vi "Hi-Tec_Voltage_calculator.vi"(0 "Carrier_1 Q (l/min)":dbl=20.0 format="%.2f", 2 "Mode":enum16{"Control Hi-Tec", "Check Hi-Tec Demands"}(ring), 5 "Carrier_2 Q (l/min)":dbl=20.0 format="%.2f", 7 "Trace Q (l/min)":dbl=20.0 format="%.2f", 9 "Release temp (deg C)":dbl=20.0 format="%.2f", 11 "Atmos Pres (mbars)":dbl=1000.0 format="%.2f", 12 "Carrier Info":string) -> (4 "Carrier 1 Voltage":dbl format="%.3f", 6 "Carrier 2 Voltage":dbl format="%.2f", 8 "Trace Voltage":dbl format="%.2f", 10 "Flowrates (kg/min)":dbl[](array[numeric]) format="%.2f", 14 "Trace_2 Voltage":dbl format="%.2f", 15 "Error Comments":string)   [LabVIEW 2015]
uses:
  Anemometry/Anemometry Sub Vis/Globals/Gas_management_global.vi
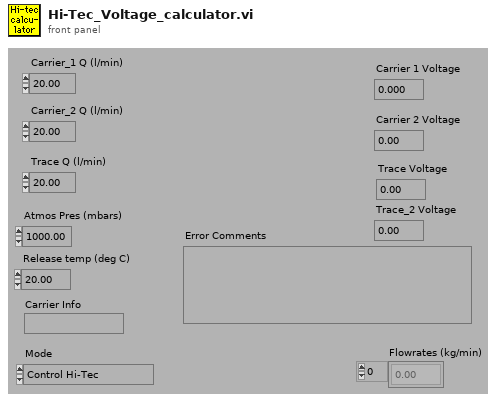
[diagram p1: front panel]
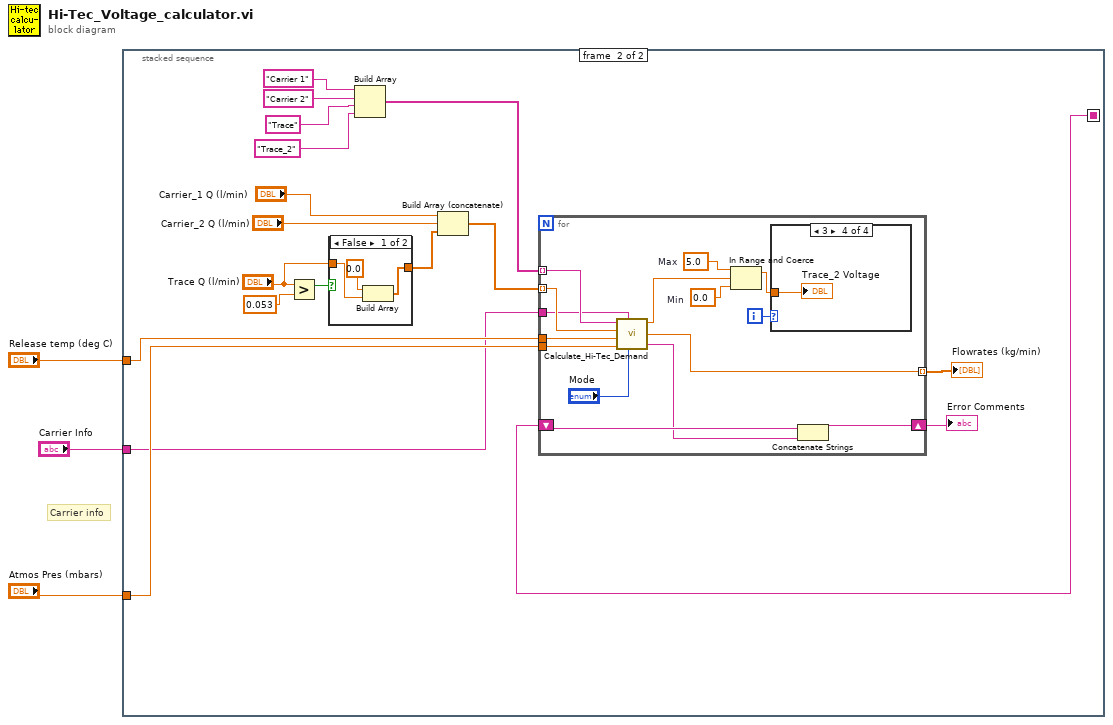
[diagram p0: block diagram]
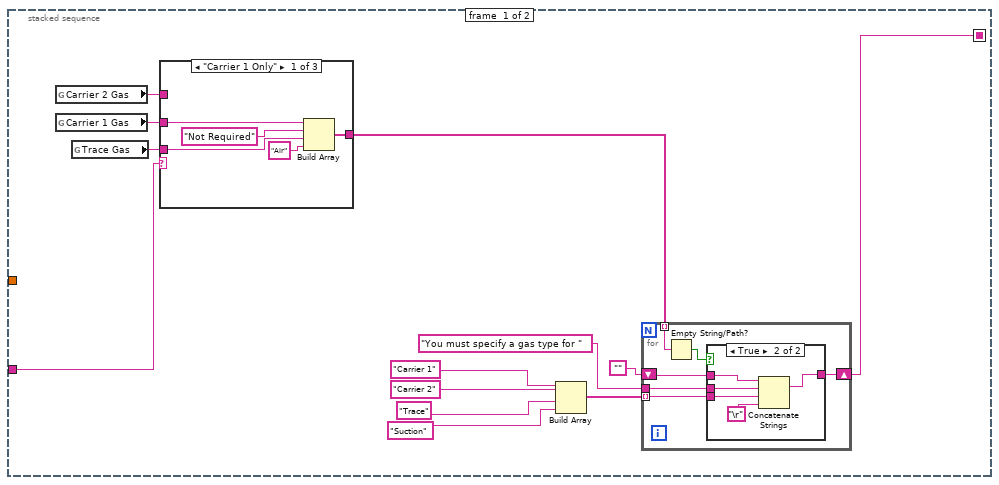
[diagram p2: hidden frame]
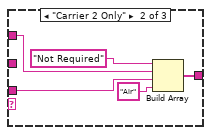
[diagram p4: hidden frame]
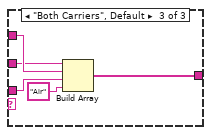
[diagram p5: hidden frame]
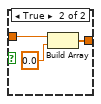
[diagram p6: hidden frame]
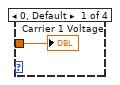
[diagram p7: hidden frame]
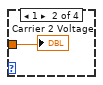
[diagram p8: hidden frame]
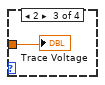
[diagram p9: hidden frame]
diagram:
  # "Carrier info"
  n1 = stacked-sequence {
    seq-local: [w6 _] -> [_ w58]
    tunnel: "Release temp (deg C)" -> [_ w60]
    tunnel: "Atmos Pres (mbars)" -> [_ w61]
    tunnel: "Carrier Info" -> [w4 w56]
    frame #0 {
      n2 = global read "Gas_management_global.vi" "Carrier 2 Gas"() -> (w14:string)
      n3 = global read "Gas_management_global.vi" "Carrier 1 Gas"() -> (w16:string)
      n4 = global read "Gas_management_global.vi" "Trace Gas"() -> (w15:string)
      n5 = case shown="\"Carrier 1 Only\"" w4 {
        tunnel: [w31 w36 w42] -> w7
        tunnel: w16 -> [w30 _ w39]
        tunnel: w15 -> [w29 w34 w41]
        tunnel: w14 -> [_ w35 w40]
        frame "Carrier 1 Only" {
          n6 = Build Array(w30, "Not Required" ("Input Element"), w29, "Air") -> (w31:string[])
        }
        frame "Carrier 2 Only" {
          n7 = Build Array("Not Required" ("Input Element"), w35, w34, "Air") -> (w36:string[])
        }
        frame "Both Carriers", Default {
          n8 = Build Array(w39, w40, w41, "Air") -> (w42:string[])
        }
      }
      n9 = Build Array("Carrier 1" ("Gas Line Name"), "Carrier 2" ("Gas Line Name"), "Trace" ("Gas Line Name"), "Suction" ("Gas Line Name")) -> (w13:string[])
      n10 = for {
        shift-right: [w18] -> w6
        shift-left: "" -> [w19]
        tunnel: "You must specify a gas type for " -> [w21]
        tunnel: w13 -> [w20] mode=indexing
        tunnel: w7 -> [w17] mode=indexing
        n11 = Empty String/Path?(string/path=w17) -> (empty?=w22:bool)
        n12 = case shown="True" w22 {
          tunnel: w21 -> [_ w28]
          tunnel: w20 -> [_ w27]
          tunnel: w19 -> [w23 w26]
          tunnel: [w23 w25] -> w18
          frame False {
          }
          frame True {
            n13 = Concatenate Strings(w26, w28, w27, "\r") -> (w25:string)
          }
        }
      }
    }
    frame #1 {
      n14 = Greater?(x="Trace Q (l/min)", y=0.053) -> (0:w46:bool)
      n15 = case shown="False" w46 {
        tunnel: "Trace Q (l/min)" -> [w63 w67]
        tunnel: [w64 w65] -> w44
        frame False {
          n16 = Build Array(0.0 ("element"), w63) -> (w64:dbl[])
        }
        frame True {
          n17 = Build Array(w67, 0.0 ("element")) -> (w65:dbl[])
        }
      }
      n18 = Build Array("Carrier 1" ("Gas Line Name"), "Carrier 2" ("Gas Line Name"), "Trace" ("Gas Line Name"), "Trace_2" ("Gas Line Name")) -> (w51:string[])
      n19 = Build Array (concatenate)("Carrier_1 Q (l/min)", "Carrier_2 Q (l/min)", w44) -> (w50:dbl[])
      n20 = for {
        shift-right: [w79] -> w57
        shift-left: w58 -> [w81]
        tunnel: w61 -> [w78]
        tunnel: w60 -> [w77]
        tunnel: w50 -> [w76] mode=indexing
        tunnel: [w70] -> w59 mode=indexing
        tunnel: w51 -> [w75] mode=indexing
        tunnel: w56 -> [w68]
        i -> [w82]
        w72 = 0.0  # Min
        w73 = 5.0  # Max
        n21 = call "Calculate_Hi-Tec_Demand.vi"("Gas Line Name"=w75, "Carrier Info"=w68, "Flowrate"=w76, "Release temp (deg C)"=w77, "Mode"="Mode", "Atmos Pres (mbars)"=w78) -> ("Demand Voltage"=w71:dbl, "Flowrate (kg/min)"=w70:dbl, "Error messages"=w80:string)
        n22 = In Range and Coerce(upper limit=w73, x=w71, lower limit=w72) -> (coerced(x)=w69:dbl)  [unwired: 1 out]
        n23 = case shown="3" w82 {
          tunnel: w69 -> [w83 w84 w85 w86]
          frame 0, Default {
            "Carrier 1 Voltage" <- w83
          }
          frame 1 {
            "Carrier 2 Voltage" <- w84
          }
          frame 2 {
            "Trace Voltage" <- w85
          }
          frame 3 {
            "Trace_2 Voltage" <- w86
          }
        }
        n24 = Concatenate Strings(w81, w80) -> (w79:string)
      }
      "Flowrates (kg/min)" <- w59
      "Error Comments" <- w57
    }
  }
